vi "ShiftFrame (SubVI).vi"(8 "Y shift":sgl, 9 "X shift":sgl, 11 "Application in":refnum<vi>) -> (3 "Application out":refnum<vi>)   [LabVIEW 2014]
uses:
  <userlib>/Nanonis Prog Interface V5/Nanonis Prog Interface.lvlib
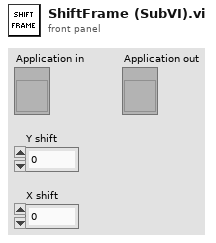
[diagram p1: front panel]
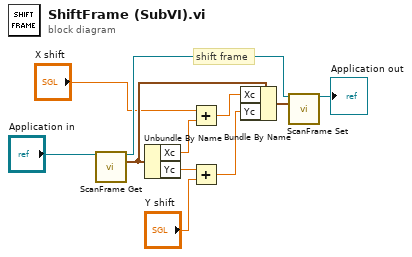
[diagram p0: block diagram]
diagram:
  # "shift frame"
  n1 = call <userlib>:"ScanFrame Get.vi"("Application ref in"="Application in") -> ("Application ref out"=w10:refnum<vi>, "Center coordinates (m)"=w11:cluster{"Xc":sgl, "Yc":sgl})  [unwired: 10 in, 3 out]
  n2 = Unbundle By Name(w11) -> ("Xc"=w1:sgl, "Yc"=w5:sgl)
  n3 = Add(x="X shift", y=w1) -> (x+y=w4:sgl)
  n4 = Add(x=w5, y="Y shift") -> (x+y=w6:sgl)
  n5 = Bundle By Name(cluster=w11, "Xc"=w4, "Yc"=w6) -> (w3:cluster{"Xc":sgl, "Yc":sgl})
  n6 = call <userlib>:"ScanFrame Set.vi"("Application ref in"=w10, "Center coordinates (m)"=w3) -> ("Application ref out"=→"Application out":refnum<vi>)  [unwired: 12 in, 1 out]
